vi "Test Helper Loop waiting for Start.vi"(8 "error in (no error)":errorcluster, 11 "Helper Loop Test In":refnum<class "Helper Loop Test.lvclass">) -> (0 "error out":errorcluster, 3 "Helper Loop Test Out":refnum<class "Helper Loop Test.lvclass">)   [LabVIEW 2020, in "Helper Loop Test.lvclass"]
uses:
  Helper Loop Test.lvclass
  C:/Program Files (x86)/National Instruments/LabVIEW 2020/vi.lib/Astemes/LUnit/Test Case.lvclass
  source/Framework Test Suite/Mock Process/Mock Process.lvclass
  C:/git/astemes-triarc-framework/source/Framework/Process/Process.lvclass
  source/Framework/Process/Process.lvclass/Process.ctl
  <vilib>/Astemes/LUnit/Test Case.lvclass/Test Case.ctl
  source/Framework/Process/Public/Lifecycle/Get Lifecycle State.vi
  source/Framework/Process/Private/SubVIs/Wait for finish.vi
  source/Framework/Process/Private/SubVIs/Set Lifecycle State.vi
  source/Framework/Process/Protected/Messaging/Send Message.vi
  <vilib>/Astemes/LUnit/Append Fail Result.vi
  <vilib>/Astemes/LUnit/Append Pass Result.vi
  <vilib>/Utility/error.llb/Clear Errors.vi
  source/Framework/Process/Private/SubVIs/Handle Debug Data.vi
  source/Framework/Logging/Log Debug.vi
  <vilib>/AdvancedString/1D String Array to Delimited String.vi
  <vilib>/Utility/High Resolution Relative Seconds.vi
  <vilib>/Utility/error.llb/Error Cluster From Error Code.vi
  source/Framework/Process/Public/Read Name.vi
  source/Framework/Broadcast Event Dequeuers/Dequeue Broadcast Message.vi
  source/Framework/Callback/Callback.lvclass
  source/Framework/Process/Process.lvclass
  Helper Loop Test.lvclass/Helper Loop Test.ctl
  <vilib>/Astemes/LUnit/Test Case.lvclass
  source/Framework/Broadcast Event Helpers/Broadcast Event Helpers.lvlib
  C:/git/astemes-triarc-framework/source/Framework/Base/Base.lvclass
  C:/git/astemes-triarc-framework/source/Framework/Configuration File/Configuration File.lvclass
  C:/git/astemes-triarc-framework/source/Framework/Configuration/Configuration.lvclass
  C:/git/astemes-triarc-framework/source/Framework/Error Handler Interface/Error Handler Interface.lvclass
  C:/git/astemes-triarc-framework/source/Framework/Logging/Logging.lvclass
  C:/git/astemes-triarc-framework/source/Framework Test Suite/Mock Process/Mock Process.lvclass
  C:/git/astemes-triarc-framework/source/Framework/Async Handler/Async Handler.lvclass
  C:/git/astemes-triarc-framework/source/Framework/Helper Loop/Helper Loop.lvclass
  source/Framework Test Suite/Support/Test Support.lvlib
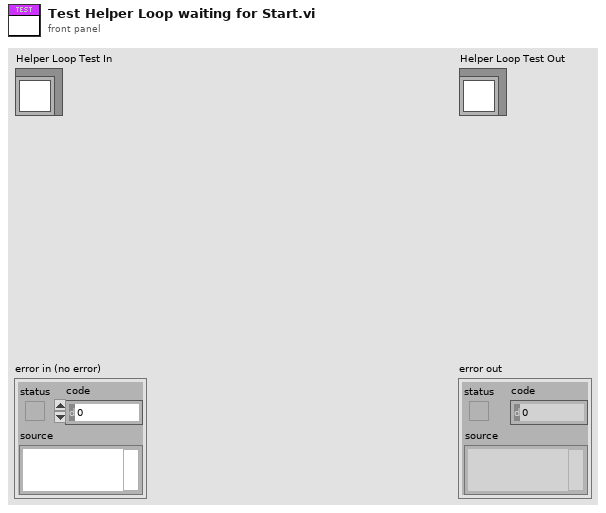
[diagram p1: front panel]
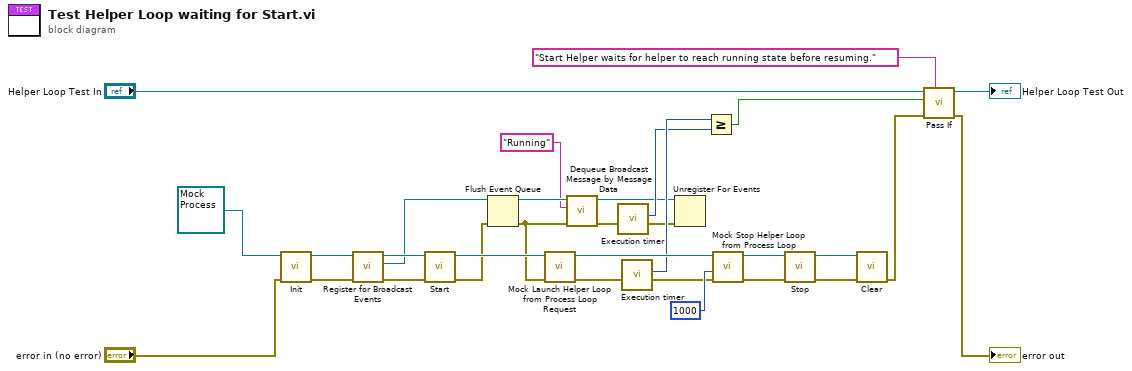
[diagram p0: block diagram]
diagram:
  n1 = call-dynamic "Init.vi"("error in (no error)"="error in (no error)", "Mock Process In"=refnum<class "Mock Process.lvclass"> refnum) -> ("error out"=w29:errorcluster, "Mock Process Out"=w30:refnum<class "Mock Process.lvclass">)  [unwired: 8 in]
  n2 = call "Register for Broadcast Events.vi"("error in (no error)"=w29, "Process In"=w30) -> ("error out"=w27:errorcluster, "Event Registration Refnum Out"=w14:refnum<event-registration>, "Process Out"=w28:refnum<class "Mock Process.lvclass">)  [unwired: 7 in]
  n3 = call "Start.vi"("error in (no error)"=w27, "Process In"=w28) -> ("error out"=w12:errorcluster, "Process Out"=w26:refnum<class "Mock Process.lvclass">)  [unwired: 7 in, 1 out]
  n4 = Flush Event Queue(0:w14, 3:w12) -> (8:w13:refnum<event-registration>, 11:w4:errorcluster)  [unwired: 4 in, 1 out]
  n5 = call "Mock Launch Helper Loop from Process Loop Request.vi"("error in (no error)"=w4, "Mock Process in"=w26) -> ("error out"=w10:errorcluster, "Mock Process out"=w25:refnum<class "Mock Process.lvclass">)  [unwired: 8 in]
  n6 = call "Dequeue Broadcast Message by Message Data.vi"("error in (no error)"=w4, "Message Data"="Running", "Event Registration Refnum"=w13) -> ("error out"=w11:errorcluster, "Event Registration Refnum Out"=w5:refnum<event-registration>)  [unwired: 4 in, 3 out]
  n7 = call "Execution timer.vi"("error in (no error)"=w11) -> ("error out"=w6:errorcluster, "Current or Duration [ms]"=w7:u32)  [unwired: 9 in]
  n8 = call "Execution timer.vi"("error in (no error)"=w10) -> ("error out"=w9:errorcluster, "Current or Duration [ms]"=w8:u32)  [unwired: 9 in]
  n9 = Unregister For Events(event registration refnum=w5, error in=w6) -> ()  [unwired: 1 out]
  n10 = Greater Or Equal?(x=w8, y=w7) -> (x >= y?=w3:bool)
  n11 = call "Mock Stop Helper Loop from Process Loop.vi"("error in (no error)"=w9, "timeout in ms (-1)"=1000, "Mock Process in"=w25) -> ("error out"=w23:errorcluster, "Mock Process out"=w24:refnum<class "Mock Process.lvclass">)  [unwired: 6 in, 1 out]
  n12 = call "Stop.vi"("error in (no error)"=w23, "Process In"=w24) -> ("error out"=w22:errorcluster, "Process Out"=w1:refnum<class "Mock Process.lvclass">)  [unwired: 7 in, 1 out]
  n13 = call-dynamic "Clear.vi"("error in (no error)"=w22, "Mock Process In"=w1) -> ("error out"=w21:errorcluster)  [unwired: 9 in]
  n14 = call <vilib>:"Pass If.vi"("Description"="Start Helper waits for helper to reach running state before resuming.", "error in (no error)"=w21, "Pass?"=w3, "LUnit Test Case In"="Helper Loop Test In") -> ("error out"=→"error out":errorcluster, "LUnit Test Case Out"=→"Helper Loop Test Out":refnum<class "Helper Loop Test.lvclass">)  [unwired: 6 in]
